vi "New plot1.vi"() -> (0 "Closed w":bool)   [LabVIEW 2022 SP3]
uses:
  <vilib>/Analysis/1siggen.llb/Ramp Pattern by Samples.vi
  <vilib>/Analysis/NI_AALBase.lvlib
  <vilib>/gmath/NI_Gmath.lvlib
panel:
  in  "Tab Control":enum32{"Graph", "Information"}(tab)
  out "Waveform Graph":waveform(dbl)[](graph) caption="Waveform Graph 2"
  in  "Local Mode":enum32{"Resume", "Hold"}(radio)
  in  "Refresh time":u32
  out "Filename":string
  out "Trace name":string
  out "Mode signal_Global":string
  out "Execution:State":T1(ring)
  out "total \nrefresh time":u32
  out "message":string
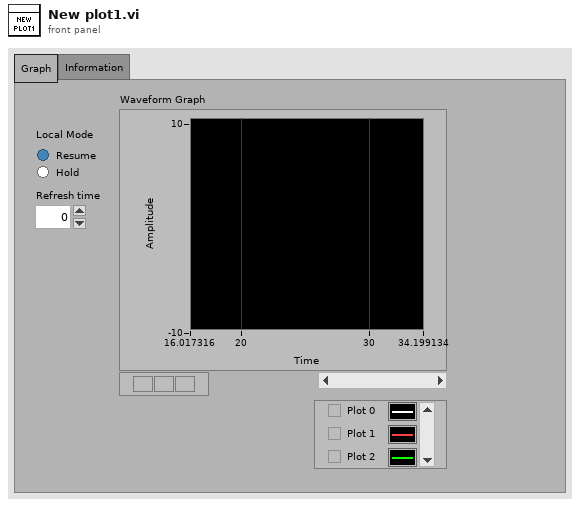
[diagram p1: front panel]
types:
  T1 = enum32{"Bad", "Idle", "Run top level", "Running"}
  T2 = cluster{"plot Names":string[], "Waveforms arrays":waveform(dbl)[], "signals_HW":string[][], "Waveforms arrays csv":waveform(dbl)[], "signals_csv":string[], "Signals_name":string[], "Mode_signal_conf":u8, "Request_plots_array":cluster{string, waveform(dbl)}[], "time out":i32, " global r time":u32}
  T3 = enum32{"Invalid", "Standard", "Closed", "Hidden", "Minimized", "Maximized"}
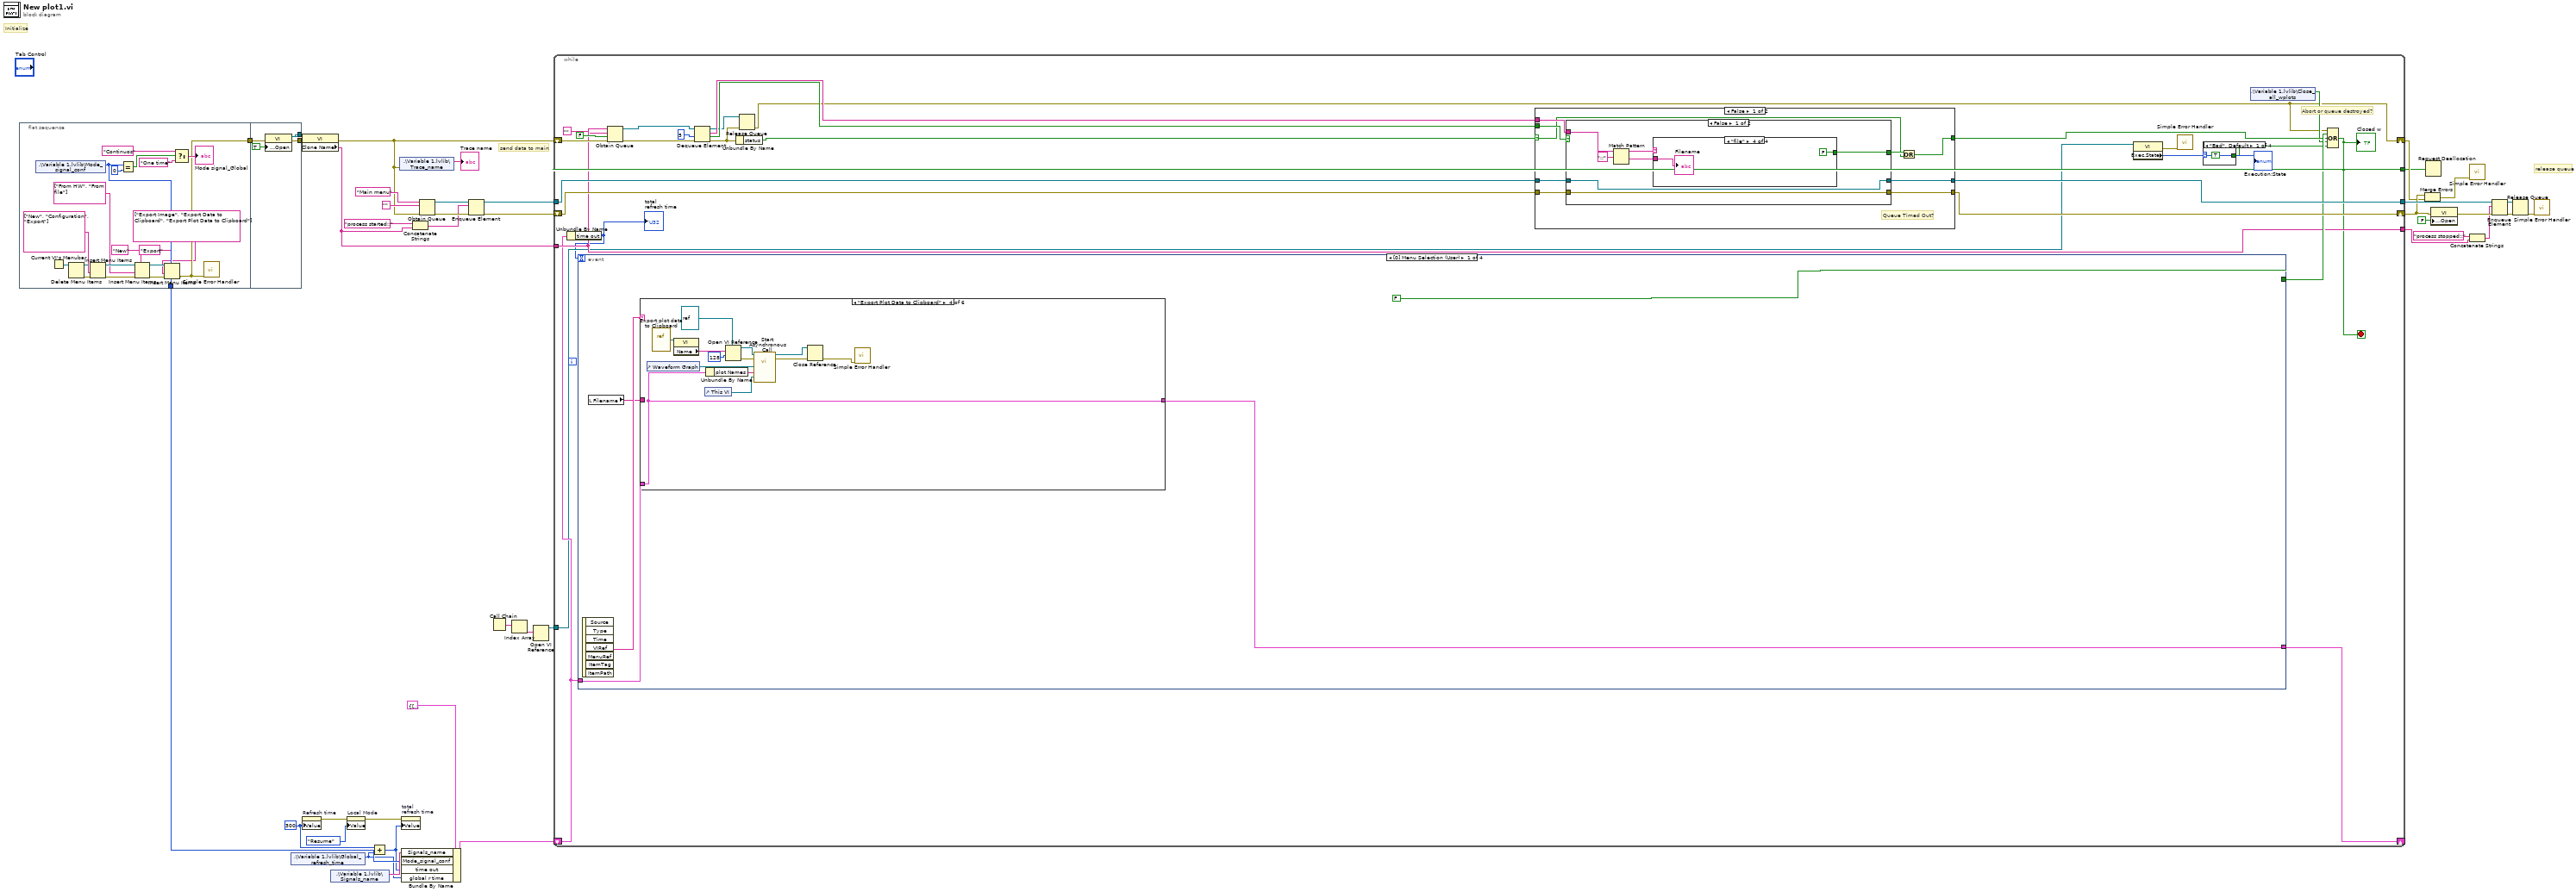
[diagram p0: block diagram]
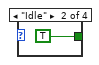
[diagram p2: hidden frame]
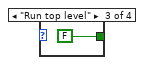
[diagram p3: hidden frame]
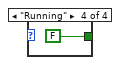
[diagram p4: hidden frame]
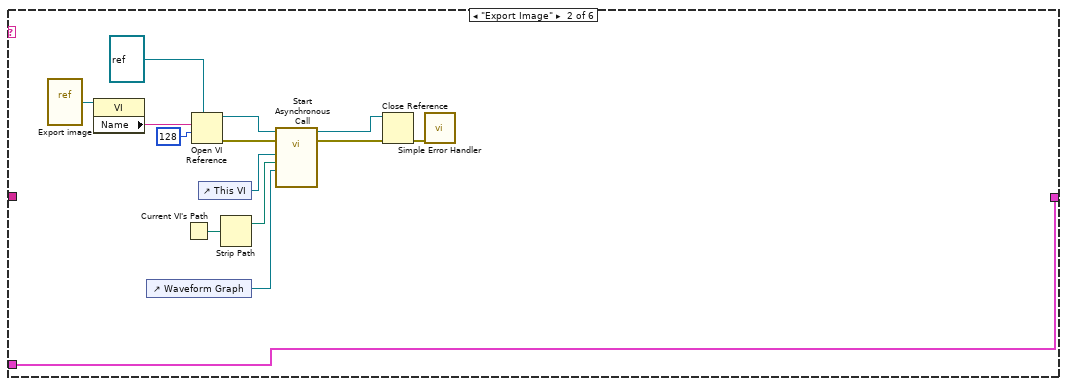
[diagram p6: hidden frame]
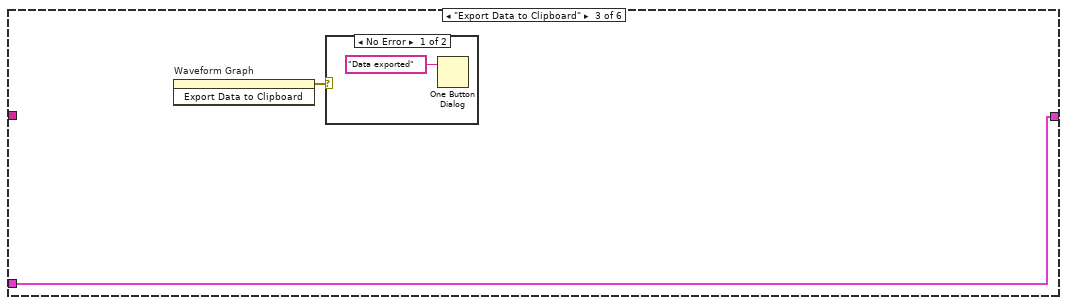
[diagram p7: hidden frame]
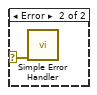
[diagram p8: hidden frame]
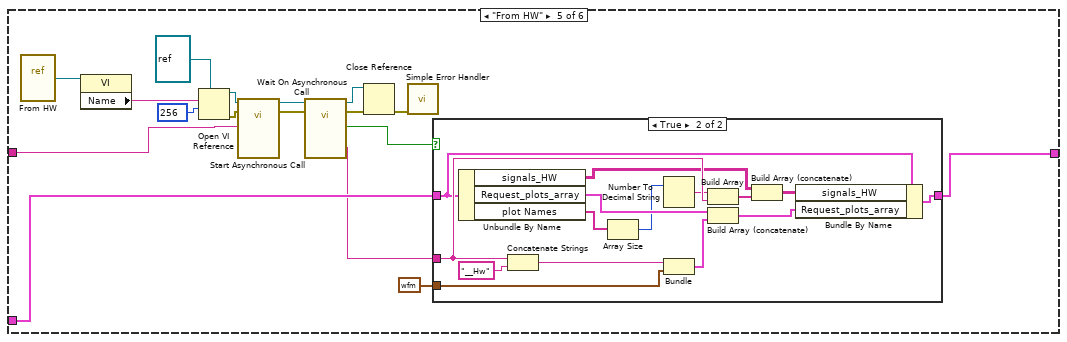
[diagram p9: hidden frame]
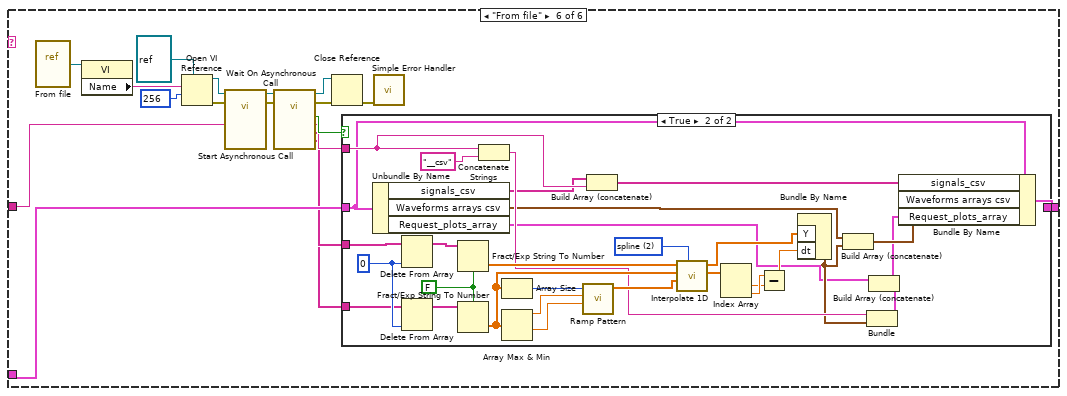
[diagram p11: hidden frame]
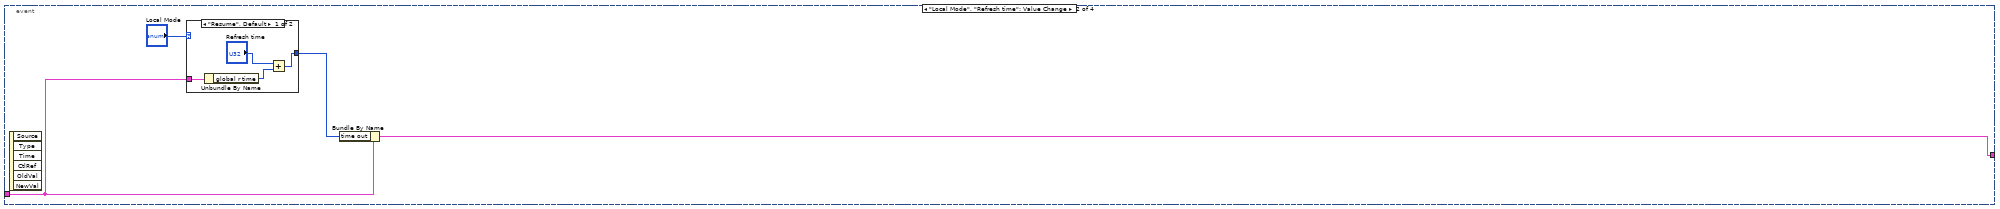
[diagram p13: hidden frame]
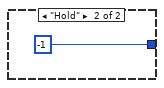
[diagram p14: hidden frame]
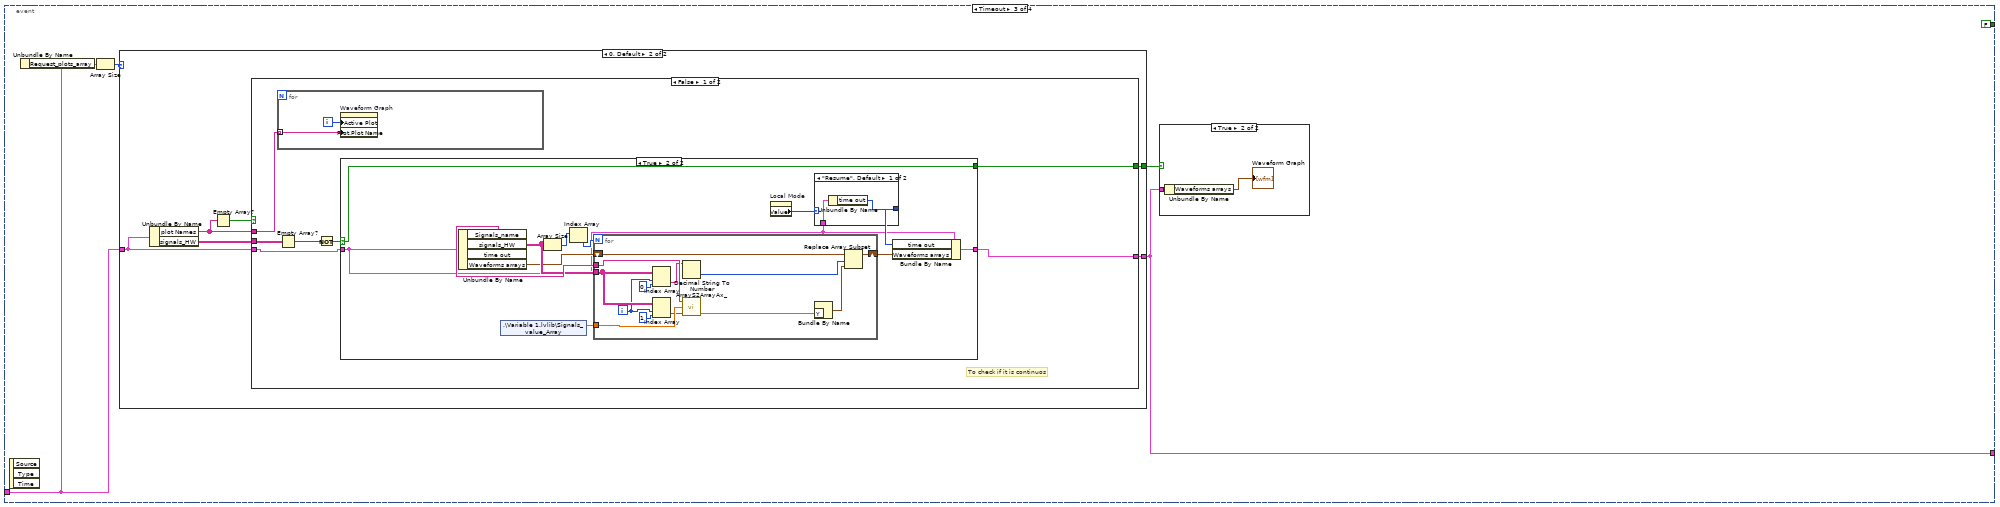
[diagram p15: hidden frame]
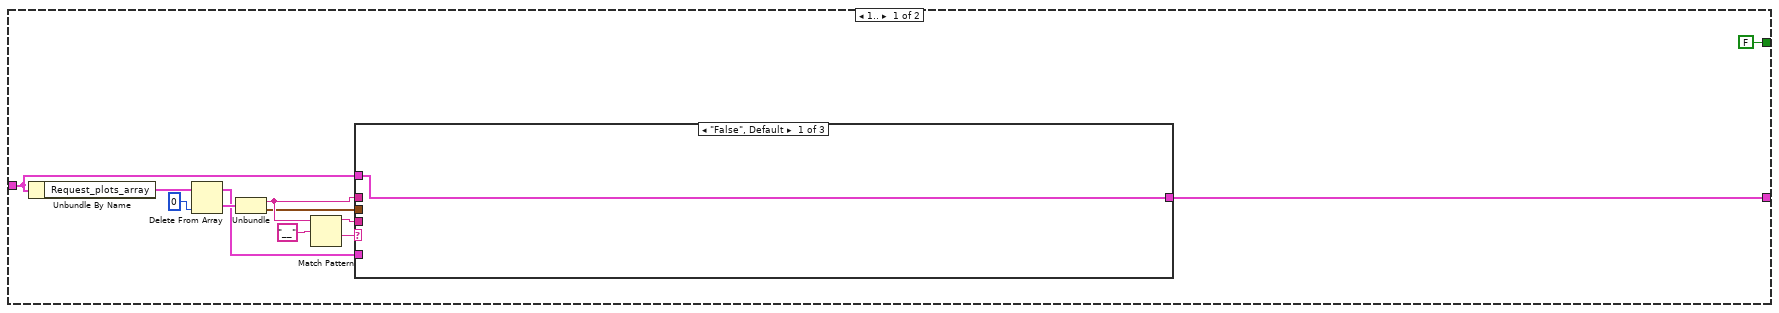
[diagram p17: hidden frame]
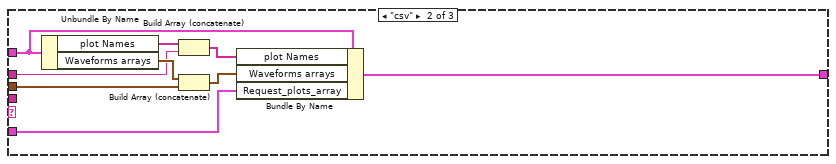
[diagram p18: hidden frame]
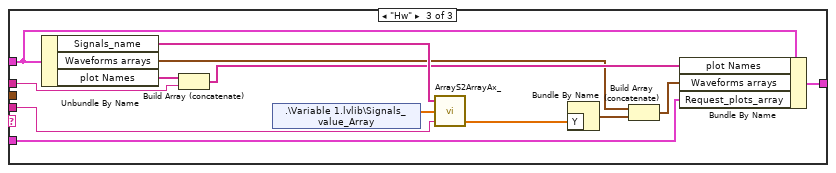
[diagram p19: hidden frame]
diagram:
  w5 = u32 300 ("Refresh time")
  # "Initialize"
  # "send data to main"
  # "release queue"
  n1 = flat-sequence {
    tunnel: [w46] -> w12
    tunnel: [w43] -> w1
    tunnel: [w62] -> w19
    tunnel: [w61] -> w34
    tunnel: w1 -> [w60]
    frame #0 {
      n2 = shared-variable ".\\Variable 1.lvlib\\Mode_signal_conf"() -> (w46:u8)  [unwired: 1 in, 1 out]
      n3 = Current VI's Menubar() -> (w54:refnum<k9>)
      n4 = Delete Menu Items(9:w54) -> (0:w53:errorcluster, 3:w52:refnum<k9>)  [unwired: 3 in]
      n5 = Insert Menu Items(6:w53, 7:string[] ["New", "Configuration", "Export"], 9:w52) -> (0:w59:errorcluster, 3:w58:refnum<k9>)  [unwired: 3 in, 1 out]
      n6 = Equal?(x=w46, y=u8 0) -> (x = y?=w50:bool)
      n7 = Insert Menu Items(5:"New", 6:w59, 7:string[] ["From HW", "From file"], 9:w58) -> (0:w45:errorcluster, 3:w44:refnum<k9>)  [unwired: 2 in, 1 out]
      n8 = Insert Menu Items(5:"Export" ("menu tag"), 6:w45, 7:string[] ["Export Image", "Export Data to Clipboard", "Export Plot Data to Clipboard"], 9:w44) -> (0:w43:errorcluster)  [unwired: 2 in, 2 out]
      n9 = Select(t="Continuos", s=w50, f="One time") -> (s? t:f=→"Mode signal_Global":string)
      n10 = call <vilib>:"Simple Error Handler.vi"("error in (no error)"=w43) -> ()  [unwired: 4 in, 5 out]
    }
    frame #1 {
      n11 = property class="VI"(error in=w60, "Front Panel.Open"=TRUE ("Front Panel Window:Open")) -> (reference out=w62:refnum<vi>, error out=w61:errorcluster)  [unwired: 1 in]
    }
  }
  n12 = shared-variable ".\\Variable 1.lvlib\\Global_refresh_time"() -> (w2:u16)  [unwired: 1 in, 1 out]
  n13 = property class="VI"(reference=w19, error in=w34) -> (error out=w10:errorcluster, "Clone Name"=w11:string)  [unwired: 1 out]
  n14 = property on="Refresh time" class="DigNum (strict)"("Value"=w5) -> (error out=w8:errorcluster)  [unwired: 2 in, 1 out]
  n15 = shared-variable ".\\Variable 1.lvlib\\Signals_name"() -> (w13:string[])  [unwired: 1 in, 1 out]
  n16 = property on="Local Mode" class="RadioBtnsControl (strict)"(error in=w8, "Value"=enum32{"Resume", "Hold"}."Resume" ("Local Mode")) -> (error out=w4:errorcluster)  [unwired: 1 in, 1 out]
  n17 = Add(x=w5, y=w2) -> (x+y=w3:u32)
  n18 = shared-variable ".\\Variable 1.lvlib\\Trace_name"(error in=w10) -> (→"Trace name":string)  [unwired: 1 out]
  n19 = property on="total \nrefresh time" class="DigNum (strict)"(error in=w4, "Value"=w3) -> ()  [unwired: 1 in, 2 out]
  n20 = Bundle By Name(cluster=T2 {"plot Names"=[], "Waveforms arrays"=[], "signals_HW"=[], "Waveforms arrays csv"=[], "signals_csv"=[], "Signals_name"=[], "Mode_signal_conf"=0, "Request_plots_array"=[], "time out"=300, " global r time"=0}, "Signals_name"=w13, "Mode_signal_conf"=w12, "time out"=w3, "global r time"=w2) -> (w14:T2)
  n21 = Concatenate Strings("process started::" ("name (unnamed)"), w11) -> (w35:string)
  n22 = Obtain Queue(name (unnamed)="Main menu", element data type="", error in (no error)=w10) -> (queue out=w37:refnum<queue>, error out=w36:errorcluster)  [unwired: 2 in, 1 out]
  n23 = Enqueue Element(queue=w37, element=w35, error in (no error)=w36) -> (queue out=w33:refnum<queue>, error out=w32:errorcluster)  [unwired: 1 in, 1 out]
  n24 = Call Chain() -> (call chain=w18:string[])
  n25 = Index Array(array=w18) -> (element=w17:string)  [unwired: 1 in]
  n26 = Open VI Reference(vi path=w17) -> (vi reference=w16:refnum<vi>)  [unwired: 5 in, 1 out]
  n27 = while {
    tunnel: w33 -> [w91]
    tunnel: [w89] -> w31
    shift-right: [w88] -> w25
    shift-left: w32 -> [w90]
    shift-right: [w64] -> w24
    shift-left: w10 -> [w81]
    tunnel: [w73] -> w21
    tunnel: w16 -> [w69]
    tunnel: w11 -> [w73]
    shift-right: [w74] -> _
    shift-left: w14 -> [w72]
    tunnel: [w66] -> w7
    stop <- w66 stop-if-true
    # "Abort or queue destroyed?"
    n28 = Unbundle By Name(w72) -> ("time out"=w65:i32)
    "total \nrefresh time" <- w65
    n29 = event shown="[0] Menu Selection (User)" {
      selector: _ -> [_ _ _ _]
      dyn-events: _ -> [_ _ _ _]
      timeout: w65 -> [_ _ _ _]
      tunnel: [FALSE _ FALSE w318] -> w77
      tunnel: [w97 w218 w226 _] -> w74
      tunnel: w72 -> [w98 w216 w229 _]
      event Menu Selection (User) {
        n30 = event-data() -> ("ItemTag"=w100:string)  [unwired: 1 in, 6 out]
        n31 = local read "Filename"() -> (w96:string)
        n32 = case shown="\"Export Plot Data to Clipboard\"" w100 {
          tunnel: [w101 w115 w117 w126 w144 w176] -> w97
          tunnel: w98 -> [w101 w115 w117 w126 w135 w177]
          tunnel: w96 -> [_ _ _ _ w136 w166]
          frame "False", Default {
          }
          frame "Export Image" {
            n33 = vi-ref "Export image.vi"() -> (w109:refnum<vi>)
            n34 = property class="VI"(reference=w109) -> ("Name"=w111:string)  [unwired: 1 in, 2 out]
            n35 = control-ref of="Waveform Graph"() -> (w104:refnum<vi>)
            n36 = Current VI's Path() -> (path=w114:path)
            n37 = Open VI Reference(type specifier VI Refnum (for type only)=refnum<vi> refnum ("reference"), vi path=w111, options=128) -> (vi reference=w112:refnum<vi>, error out=w113:errorcluster)  [unwired: 3 in]
            n38 = control-ref of="This VI"() -> (w107:refnum<vi>)
            n39 = Strip Path(path=w114) -> (stripped path=w106:path)  [unwired: 1 out]
            n40 = call-by-ref "Start Asynchronous Call"(reference=w112, error in=w113, "Graph reference"=w104, "Folder selection"=w106, "VI caller"=w107) -> (reference out=w103:refnum<vi>, error out=w102:errorcluster)  [unwired: 8 in, 1 out]
            n41 = Close Reference(reference=w103, error in (no error)=w102) -> (error out=w105:errorcluster)
            n42 = call <vilib>:"Simple Error Handler.vi"("error in (no error)"=w105) -> ()  [unwired: 4 in, 5 out]
          }
          frame "Export Data to Clipboard" {
            n43 = invoke on="Waveform Graph" class="WFGraph (strict)" method="Export Data to Clipboard"() -> (error out=w116:errorcluster)  [unwired: 3 in, 2 out]
            n44 = case shown="No Error" w116 {
              selector: w116 -> [_ w119]
              frame No Error {
                n45 = One Button Dialog(message="Data exported") -> ()  [unwired: 1 in, 1 out]
              }
              frame Error {
                n46 = call <vilib>:"Simple Error Handler.vi"("error in (no error)"=w119) -> ()  [unwired: 4 in, 5 out]
              }
            }
          }
          frame "Export Plot Data to Clipboard" {
            n47 = control-ref of="Waveform Graph"() -> (w125:refnum<vi>)
            n48 = vi-ref "Export plot data to Clipboard.vi"() -> (w121:refnum<vi>)
            n49 = property class="VI"(reference=w121) -> ("Name"=w132:string)  [unwired: 1 in, 2 out]
            n50 = control-ref of="This VI"() -> (w120:refnum<vi>)
            n51 = Unbundle By Name(w126) -> ("plot Names"=w128:string[])
            n52 = Open VI Reference(type specifier VI Refnum (for type only)=refnum<vi> refnum ("reference"), vi path=w132, options=128) -> (vi reference=w131:refnum<vi>, error out=w130:errorcluster)  [unwired: 3 in]
            n53 = call-by-ref "Start Asynchronous Call"(reference=w131, error in=w130, "VI caller"=w120, "List Plots"=w128, "Graph reference"=w125) -> (reference out=w123:refnum<vi>, error out=w122:errorcluster)  [unwired: 2 in, 1 out]
            n54 = Close Reference(reference=w123, error in (no error)=w122) -> (error out=w124:errorcluster)
            n55 = call <vilib>:"Simple Error Handler.vi"("error in (no error)"=w124) -> ()  [unwired: 4 in, 5 out]
          }
          frame "From HW" {
            n56 = vi-ref "From HW.vi"() -> (w145:refnum<vi>)
            n57 = property class="VI"(reference=w145) -> ("Name"=w137:string)  [unwired: 1 in, 2 out]
            n58 = Open VI Reference(type specifier VI Refnum (for type only)=refnum<vi> refnum ("reference"), vi path=w137, options=256) -> (vi reference=w146:refnum<vi>, error out=w149:errorcluster)  [unwired: 3 in]
            n59 = call-by-ref "Start Asynchronous Call"(reference=w146, error in=w149, "Plot window"=w136) -> (reference out=w142:refnum<vi>, error out=w143:errorcluster)  [unwired: 2 in, 3 out]
            n60 = call-by-ref "Wait On Asynchronous Call"(reference=w142, error in=w143) -> (reference out=w141:refnum<vi>, error out=w140:errorcluster, "Y name"=w133:string, "Ready?"=w139:bool)  [unwired: 3 in, 1 out]
            n61 = Close Reference(reference=w141, error in (no error)=w140) -> (error out=w148:errorcluster)
            n62 = call <vilib>:"Simple Error Handler.vi"("error in (no error)"=w148) -> ()  [unwired: 4 in, 5 out]
            n63 = case shown="True" w139 {
              tunnel: w133 -> [_ w164]
              tunnel: [w150 w159] -> w144
              tunnel: w135 -> [w150 w163]
              tunnel: waveform(dbl) {"t0"=timestamp(0 s since 1904-01-01), "dt"=1.0, "Y"=[]} ("Waveform") -> [_ w157]
              frame False {
              }
              frame True {
                n64 = Unbundle By Name(w163) -> ("signals_HW"=w162:string[][], "Request_plots_array"=w156:cluster{string, waveform(dbl)}[], "plot Names"=w153:string[])
                n65 = Concatenate Strings(w164, "__Hw" ("string")) -> (w158:string)
                n66 = Array Size(array=w153) -> (size(s)=w152:i32)
                n67 = Number To Decimal String(number=w152) -> (decimal integer string=w151:string)  [unwired: 1 in]
                n68 = Bundle(w158, "Waveform"=w157) -> (w155:cluster{string, "Waveform":waveform(dbl)})  [unwired: 1 in]
                n69 = Build Array(w151, w164) -> (w161:string[])
                n70 = Build Array (concatenate)(w156, w155) -> (w154:cluster{string, "Waveform":waveform(dbl)}[])
                n71 = Build Array (concatenate)(w162, w161) -> (w160:string[][])
                n72 = Bundle By Name(cluster=w163, "signals_HW"=w160, "Request_plots_array"=w154) -> (w159:T2)
              }
            }
          }
          frame "From file" {
            n73 = vi-ref "From file.vi"() -> (w180:refnum<vi>)
            n74 = property class="VI"(reference=w180) -> ("Name"=w174:string)  [unwired: 1 in, 2 out]
            n75 = Open VI Reference(type specifier VI Refnum (for type only)=refnum<vi> refnum, vi path=w174, options=256) -> (vi reference=w178:refnum<vi>, error out=w183:errorcluster)  [unwired: 3 in]
            n76 = call-by-ref "Start Asynchronous Call"(reference=w178, error in=w183, "Plot window"=w166) -> (reference out=w175:refnum<vi>, error out=w173:errorcluster)  [unwired: 3 in, 4 out]
            n77 = call-by-ref "Wait On Asynchronous Call"(reference=w175, error in=w173) -> (reference out=w168:refnum<vi>, error out=w167:errorcluster, "Y subarray"=w169:string[], "X subarray"=w170:string[], "Curve name"=w171:string, "Ready?"=w172:bool)  [unwired: 4 in]
            n78 = Close Reference(reference=w168, error in (no error)=w167) -> (error out=w182:errorcluster)
            n79 = case shown="True" w172 {
              tunnel: w170 -> [_ w214]
              tunnel: w169 -> [_ w213]
              tunnel: w171 -> [_ w196]
              tunnel: w177 -> [w184 w190]
              tunnel: [w184 w191] -> w176
              frame False {
              }
              frame True {
                w205 = 2 items=["nearest", "linear", "spline", "cubic Hermite", "Lagrange"] ("method")
                w210 = FALSE ("use system decimal point (T)")
                w215 = 0 ("index")
                n80 = Unbundle By Name(w190) -> ("signals_csv"=w188:string[], "Waveforms arrays csv"=w189:waveform(dbl)[], "Request_plots_array"=w187:cluster{string, waveform(dbl)}[])
                n81 = Delete From Array(array=w214, index=w215) -> (array with subset deleted=w211:string[])  [unwired: 1 in, 1 out]
                n82 = Delete From Array(array=w213, index=w215) -> (array with subset deleted=w212:string[])  [unwired: 1 in, 1 out]
                n83 = Fract/Exp String To Number(use system decimal point (T)=w210, string=w211) -> (number=w202:dbl[])  [unwired: 2 in, 1 out]
                n84 = Fract/Exp String To Number(use system decimal point (T)=w210, string=w212) -> (number=w204:dbl[])  [unwired: 2 in, 1 out]
                n85 = Concatenate Strings(w196, "__csv" ("string")) -> (w195:string)
                n86 = Array Size(array=w204) -> (size(s)=w208:i32)
                n87 = Array Max & Min(array=w204) -> (max value=w207:dbl, min value=w206:dbl)  [unwired: 2 out]
                n88 = call-poly <vilib>:"Ramp Pattern.vi"("start"=w206, "end"=w207, "samples"=w208) -> ("Ramp Pattern"=w203:dbl[])  [unwired: 7 in, 1 out]
                n89 = Build Array (concatenate)(w188, w196) -> (w193:string[])
                n90 = call <vilib>:"Interpolate 1D.vi"("method"=w205, "xi"=w203, "X"=w204, "Y"=w202) -> ("xi used"=w201:dbl[], "yi"=w200:dbl[])  [unwired: 5 in, 1 out]
                n91 = Index Array(array=w201) -> (element #1=w198:dbl, element #2=w199:dbl)  [unwired: 2 in]
                n92 = Subtract(x=w199, y=w198) -> (x-y=w197:dbl)
                n93 = Bundle By Name("Y"=w200, "dt"=w197) -> (w194:waveform(dbl))  [unwired: 1 in]
                n94 = Build Array (concatenate)(w189, w194) -> (w192:waveform(dbl)[])
                n95 = Bundle(w195, w194) -> (w186:cluster{string, waveform(dbl)})  [unwired: 1 in]
                n96 = Build Array (concatenate)(w187, w186) -> (w185:cluster{string, waveform(dbl)}[])
                n97 = Bundle By Name(cluster=w190, "signals_csv"=w193, "Waveforms arrays csv"=w192, "Request_plots_array"=w185) -> (w191:T2)
              }
            }
            n98 = call <vilib>:"Simple Error Handler.vi"("error in (no error)"=w182) -> ()  [unwired: 4 in, 5 out]
          }
        }
      }
      event "Local Mode", "Refresh time": Value Change {
        n99 = event-data() -> ()  [unwired: 1 in, 6 out]
        n100 = case shown="\"Resume\", Default" "Local Mode" {
          tunnel: [w220 -1 ("time out")] -> w219
          tunnel: w216 -> [w223 _]
          frame "Resume", Default {
            n101 = Unbundle By Name(w223) -> ("global r time"=w221:u32)
            n102 = Add(x="Refresh time", y=w221) -> (x+y=w220:u32)
          }
          frame "Hold" {
          }
        }
        n103 = Bundle By Name(cluster=w216, "time out"=w219) -> (w218:T2)
      }
      event Timeout {
        n104 = event-data() -> ()  [unwired: 1 in, 3 out]
        n105 = Unbundle By Name(w229) -> ("Request_plots_array"=w228:cluster{string, waveform(dbl)}[])
        n106 = Array Size(array=w228) -> (size(s)=w227:i32)
        n107 = case shown="0, Default" w227 {
          tunnel: w229 -> [w240 w271]
          tunnel: [w241 w270] -> w226
          tunnel: [FALSE w268] -> w225
          frame 1.. {
            n108 = Unbundle By Name(w240) -> ("Request_plots_array"=w235:cluster{string, waveform(dbl)}[])
            n109 = Delete From Array(array=w235, index=0) -> (deleted portion=w236:cluster{string, waveform(dbl)}, array with subset deleted=w234:cluster{string, waveform(dbl)}[])  [unwired: 1 in]
            n110 = Unbundle(w236) -> (w238:string, w237:waveform(dbl))
            n111 = Match Pattern(string=w238, regular expression="__") -> (before substring=w242:string, after substring=w243:string)  [unwired: 1 in, 2 out]
            n112 = case shown="\"False\", Default" w243 {
              tunnel: w240 -> [w245 w254 w263]
              tunnel: w242 -> [_ _ w265]
              tunnel: w237 -> [_ w251 _]
              tunnel: w238 -> [_ w249 w262]
              tunnel: [w245 w247 w258] -> w241
              tunnel: w234 -> [_ w246 w256]
              frame "False", Default {
              }
              frame "csv" {
                n113 = Unbundle By Name(w254) -> ("plot Names"=w253:string[], "Waveforms arrays"=w252:waveform(dbl)[])
                n114 = Build Array (concatenate)(w253, w249) -> (w248:string[])
                n115 = Build Array (concatenate)(w252, w251) -> (w250:waveform(dbl)[])
                n116 = Bundle By Name(cluster=w254, "plot Names"=w248, "Waveforms arrays"=w250, "Request_plots_array"=w246) -> (w247:T2)
              }
              frame "Hw" {
                n117 = Unbundle By Name(w263) -> ("Signals_name"=w266:string[], "Waveforms arrays"=w255:waveform(dbl)[], "plot Names"=w257:string[])
                n118 = Build Array (concatenate)(w257, w262) -> (w261:string[])
                n119 = shared-variable ".\\Variable 1.lvlib\\Signals_value_Array"() -> (w267:dbl[])  [unwired: 1 in, 1 out]
                n120 = call "ArrayS2ArrayAx_.vi"("Signal_input"=w265, "Signals_value_Array"=w267, "Signals_name"=w266) -> ("Subarray 1x_out"=w264:sgl[])  [unwired: 2 out]
                n121 = Bundle By Name("Y"=w264) -> (w260:waveform(sgl))  [unwired: 1 in]
                n122 = Build Array (concatenate)(w255, w260) -> (w259:waveform(dbl)[])
                n123 = Bundle By Name(cluster=w263, "plot Names"=w261, "Waveforms arrays"=w259, "Request_plots_array"=w256) -> (w258:T2)
              }
            }
          }
          frame 0, Default {
            n124 = Unbundle By Name(w271) -> ("plot Names"=w273:string[], "signals_HW"=w269:string[][])
            n125 = Empty Array?(array=w273) -> (empty?=w272:bool)
            n126 = case shown="False" w272 {
              tunnel: w273 -> [w280 _]
              tunnel: w269 -> [w278 _]
              tunnel: w271 -> [w279 w314]
              tunnel: [w275 w314] -> w270
              tunnel: [w274 FALSE] -> w268
              frame False {
                # "To check if it is continuos"
                n127 = for {
                  tunnel: w280 -> [w311] mode=indexing
                  i -> [w312]
                  n128 = property on="Waveform Graph" class="WFGraph (strict)"("Active Plot"=w312, "Plot.Plot Name"=w311) -> ()  [unwired: 2 in, 2 out]
                }
                n129 = Empty Array?(array=w278) -> (empty?=w277:bool)
                n130 = Not(x=w277) -> (.not. x?=w276:bool)
                n131 = case shown="True" w276 {
                  selector: w276 -> [w281 w283]
                  tunnel: w279 -> [w282 w284]
                  tunnel: [w282 w288] -> w275
                  tunnel: [w281 w283] -> w274
                  frame False {
                  }
                  frame True {
                    n132 = Unbundle By Name(w284) -> ("Signals_name"=w293:string[], "signals_HW"=w292:string[][], "Waveforms arrays"=w289:waveform(dbl)[])  [unwired: 1 out]
                    n133 = shared-variable ".\\Variable 1.lvlib\\Signals_value_Array"() -> (w294:dbl[])  [unwired: 1 in, 1 out]
                    n134 = Array Size(array=w292) -> (size(s)=w291:i32[])
                    n135 = Index Array(array=w291) -> (element=w290:i32)  [unwired: 1 in]
                    n136 = for {
                      N: w290 -> [_]
                      tunnel: w292 -> [w308]
                      tunnel: w294 -> [w310]
                      tunnel: w293 -> [w309]
                      shift-right: [w298] -> w285
                      shift-left: w289 -> [w303]
                      i -> [w300]
                      n137 = Index Array(array=w308, index (row)=w300, index (col)=0 ("disabled index (row)")) -> (element=w306:string)
                      n138 = Index Array(array=w308, index (row)=w300, index (col)=1 ("index")) -> (element=w307:string)
                      n139 = Decimal String To Number(string=w306) -> (number=w302:i32)  [unwired: 2 in, 1 out]
                      n140 = call "ArrayS2ArrayAx_.vi"("Signal_input"=w307, "Signals_value_Array"=w310, "Signals_name"=w309) -> ("Subarray 1x_out"=w305:sgl[])  [unwired: 2 out]
                      n141 = Bundle By Name("Y"=w305) -> (w304:waveform(sgl))  [unwired: 1 in]
                      n142 = Replace Array Subset(array=w303, new element=w304, index=w302) -> (w298:waveform(dbl)[])
                    }
                    n143 = property on="Local Mode" class="RadioBtnsControl (strict)"() -> ("Value"=w287:enum32{"Resume", "Hold"})  [unwired: 2 in, 2 out]
                    n144 = case shown="\"Resume\", Default" w287 {
                      tunnel: [w295 -1 ("time out")] -> w286
                      tunnel: w284 -> [w296 _]
                      frame "Resume", Default {
                        n145 = Unbundle By Name(w296) -> ("time out"=w295:i32)
                      }
                      frame "Hold" {
                      }
                    }
                    n146 = Bundle By Name(cluster=w284, "time out"=w286, "Waveforms arrays"=w285) -> (w288:T2)
                  }
                }
              }
              frame True {
              }
            }
          }
        }
        n147 = case shown="True" w225 {
          tunnel: w226 -> [_ w231]
          frame False {
          }
          frame True {
            n148 = Unbundle By Name(w231) -> ("Waveforms arrays"=→"Waveform Graph":waveform(dbl)[])
          }
        }
      }
      event Panel Close {
        n149 = event-data() -> ()  [unwired: 1 in, 4 out]
        n150 = control-ref of="This VI"() -> (w317:refnum<vi>)
        n151 = property class="VI"(reference=w317, "FP.State"=T3."Closed" ("Front Panel Window:State")) -> (reference out=w315:refnum<vi>)  [unwired: 1 in, 1 out]
        n152 = property class="VI"(reference=w315) -> ("FP.State"=w319:T3)  [unwired: 1 in, 2 out]
        n153 = Equal?(x=w319, y=T3."Closed" ("Front Panel Window:State")) -> (x = y?=w318:bool)
      }
    }
    n154 = Obtain Queue(name (unnamed)=w73, element data type="", create if not found? (T)=FALSE, error in (no error)=w81) -> (queue out=w83:refnum<queue>, error out=w82:errorcluster)  [unwired: 1 in, 1 out]
    n155 = Dequeue Element(queue=w83, timeout in ms (-1)=5, error in (no error)=w82) -> (queue out=w79:refnum<queue>, element=w85:string, timed out?=w86:bool, error out=w78:errorcluster)
    n156 = Unbundle By Name(w78) -> ("status"=w84:bool)
    n157 = Release Queue(queue=w79, error in (no error)=w78) -> (error out=w64:errorcluster)  [unwired: 1 in, 2 out]
    n158 = case shown="False" w84 {
      selector: w84 -> [w326 w353]
      tunnel: [w325 w353] -> w76
      tunnel: w91 -> [w322 w352]
      tunnel: w90 -> [w324 w351]
      tunnel: [w321 w352] -> w89
      tunnel: [w323 w351] -> w88
      tunnel: w86 -> [w329 _]
      tunnel: w85 -> [w328 _]
      frame False {
        # "Queue Timed Out?"
        n159 = case shown="False" w329 {
          tunnel: w328 -> [w335 _]
          tunnel: [w333 FALSE] -> w327
          tunnel: w324 -> [w332 w350]
          tunnel: [w332 w350] -> w323
          tunnel: w322 -> [w331 w349]
          tunnel: [w331 w349] -> w321
          frame False {
            n160 = Match Pattern(string=w335, regular expression="::") -> (before substring=w336:string, after substring=w330:string)  [unwired: 1 in, 2 out]
            n161 = case shown="\"file\"" w336 {
              tunnel: [FALSE TRUE w342 FALSE] -> w333
              tunnel: w330 -> [_ _ w343 w345]
              frame "False", Default {
                n162 = call <vilib>:"Error Cluster From Error Code.vi"("error message (\"\")"="Invalid command received from Main VI" ("error message (\"\")"), "error code (0)"=1) -> ("error out"=w338:errorcluster)  [unwired: 7 in]
                n163 = call <vilib>:"Simple Error Handler.vi"("error in (no error)"=w338) -> ()  [unwired: 4 in, 5 out]
              }
              frame "exit" {
              }
              frame "message" {
                n164 = Equal?(x=w343, y="stop") -> (x = y?=w342:bool)
                "message" <- w343
              }
              frame "file" {
                "Filename" <- w345
              }
            }
          }
          frame True {
            n165 = Wait (ms)(milliseconds to wait=u32 10) -> ()  [unwired: 1 out]
          }
        }
        n166 = Or(x=w327, y=w326) -> (x .or. y?=w325:bool)
      }
      frame True {
      }
    }
    n167 = property class="VI"(reference=w69) -> (error out=w68:errorcluster, "Exec.State"=w71:T1)  [unwired: 1 in, 1 out]
    "Execution:State" <- w71
    n168 = call <vilib>:"Simple Error Handler.vi"("error in (no error)"=w68) -> ()  [unwired: 4 in, 5 out]
    n169 = case shown="\"Bad\", Default" w71 {
      tunnel: [TRUE ("value") TRUE ("value") FALSE ("value") FALSE ("value")] -> w70
      frame "Bad", Default {
      }
      frame "Idle" {
      }
      frame "Run top level" {
      }
      frame "Running" {
      }
    }
    n170 = shared-variable ".\\Variable 1.lvlib\\Close_all_wplots"() -> (w75:bool)  [unwired: 1 in, 1 out]
    n171 = Compound Arithmetic op=OR(w64, w77, w76, w75, w70) -> (w66:bool)
    "Closed w" <- w66
  }
  n172 = Merge Errors(w25, w24) -> (w15:errorcluster)
  n173 = Request Deallocation(w7) -> ()
  n174 = property class="VI"(error in=w25, "Front Panel.Open"=FALSE ("Front Panel Window:Open")) -> (error out=w27:errorcluster)  [unwired: 1 in, 1 out]
  n175 = call <vilib>:"Simple Error Handler.vi"("error in (no error)"=w15) -> ()  [unwired: 4 in, 5 out]
  n176 = Concatenate Strings("process stopped::" ("string"), w21) -> (w20:string)
  n177 = Enqueue Element(queue=w31, element=w20, error in (no error)=w27) -> (queue out=w30:refnum<queue>, error out=w29:errorcluster)  [unwired: 1 in, 1 out]
  n178 = Release Queue(queue=w30, error in (no error)=w29) -> (error out=w28:errorcluster)  [unwired: 1 in, 2 out]
  n179 = call <vilib>:"Simple Error Handler.vi"("error in (no error)"=w28) -> ()  [unwired: 4 in, 5 out]
